vi "Camera.v3.vi"() -> ()   [LabVIEW 2015]
uses:
  Camera Properties.ctl
  Microscope Settings.ctl
  CameraState.ctl
  ModeEnum.ctl
  Stack_State.ctl
  Stack Track.ctl
  CameraControlTypeDef.ctl
  <vilib>/DAQmx/write.llb/DAQmx Write (Analog 1D Wfm NChan NSamp).vi
  <vilib>/DAQmx/create/channels.llb/DAQmx Create Channel (AO-Voltage-Basic).vi
  <vilib>/Waveform/WDTOps.llb/WDT Number of Waveform Samples DBL.vi
  <vilib>/DAQmx/configure/timing.llb/DAQmx Timing (Sample Clock).vi
  <vilib>/DAQmx/miscellaneous.llb/DAQmx Fill In Error Info.vi
  <vilib>/vision/NI_Vision_Development_Module.lvlib
  <vilib>/DAQmx/write.llb/DAQmx Write (Digital 1D Wfm NChan NSamp).vi
panel:
  out "Relax/ms":dbl
  out "Exposure/ms":dbl
  in  "Tab Control":enum32{"Camera Settings", "Recording"}(tab)
  in  "Microscope Settings":T1={"Mode"=enum."XY", {"Scanning Mode"=12.0, "Slit Width /%"=5.0}, "Piezo Position /um"=0.0, "Exposure/ms"=40.0, "Samples per millisecond"=100.0, "Relax/ms"=10.0, "Readout Direction"=2.0, "Trigger Source"=2.0} {"Trigger Source" items=["Internal"=1.0, "External"=2.0]; "Readout Direction" items=["Forward"=1.0, "Backward"=2.0]; "?"."Scanning Mode" items=["Full Frame"=1.0, "Slit Scanning"=12.0]}
  in  "Scan":bool
  in  "Scan Continuously":bool
  out "error IO":errorcluster
  in  "V Height":dbl=2048.0 min=4.0 max=2048.0 step=4.0
  in  "V Offset":dbl min=0.0 max=0.0 step=4.0
  in  "H Offset":dbl min=0.0 max=0.0 step=4.0
  in  "H Width":dbl min=4.0 max=2048.0 step=4.0
  in  "Advanced DCAM Controls":i32(listbox) caption="Multicolumn Listbox"
  in  "Properties":T2=4211904 items=["SENSOR MODE"=4212128, "CCD MODE"=4212384, "READOUT MODE"=4211872, "ACTIVE VIEW INDEX"=4343136, "BITS PER CHANNEL"=4342976, "IMAGE PIXEL TYPE"=4343296, "BINNING"=4215968, "EXPOSURE TIME"=2049184, "CONTRAST GAIN"=3163312, "CONTRAST OFFSET"=3163328, "LIGHT MODE"=2114720, "SENSITIVITY"=2114992, "PHOTON IMAGING MODE"=2115200, "HIGH DYNAMIC RANGE MODE"=3163360, "WHITE BALANCE"=3163568, "TEMPERATURE"=2115232, "TEMPERATURE TARGET"=2115264, "SENSOR COOLER FAN"=2115296, "LINEBUNDLE HEIGHT"=4212192, "MECHANICAL SHUTTER"=2115488, "BACK FOCUS POSITION"=8422304, "TRIGGER CONNECTOR"=1066432, "TRIGGER SOURCE"=1066144, "OUTPUT TRIGGER SOURCE"=1852576, "TRIGGER GLOBAL EXPOSURE"=2049680, "FIRST TRIGGER BEHAVIOR"=2049696, "CHANNEL SYNC"=1852352, "READOUT DIRECTION"=4211904, "PRE HSYNC COUNT"=1852704, "INTERNAL LINE SPEED"=4191408, "INTERNAL LINE INVERVAL"=4191424]
  out "Waves":waveform(dbl)[](graph)
  out "Image":T3(plugin-control)
  out "Histogram":T4(graph)
  in  "stop":bool
  in  "Calibration":bool
  in  "MultiD Scan":bool
  in  "Stage Controller":bool
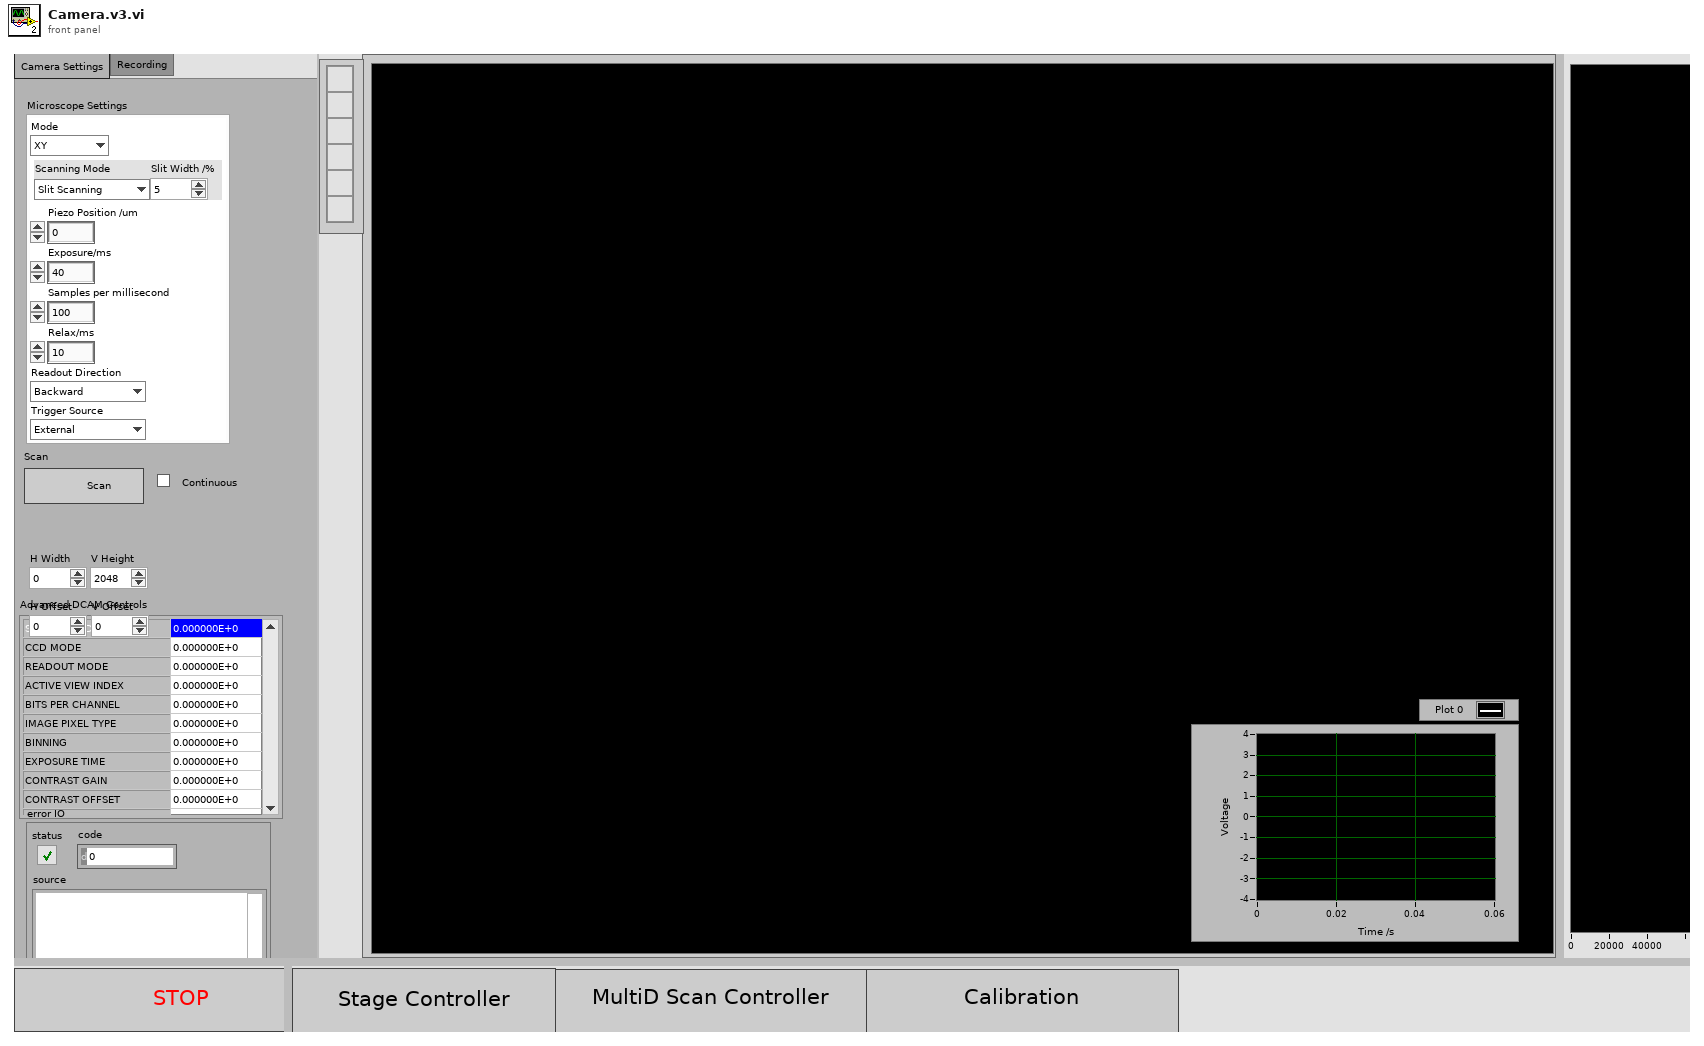
[diagram p1: front panel]
types:
  T1 = typedef "Microscope Settings.ctl" = cluster{"Mode":enum16{"X", "XY", "XYZ", "XYZT", "XYZC"}, cluster{"Scanning Mode":dbl, "Slit Width /%":dbl}, "Piezo Position /um":dbl, "Exposure/ms":dbl, "Samples per millisecond":dbl, "Relax/ms":dbl, "Readout Direction":dbl, "Trigger Source":dbl}
  T2 = typedef "Camera Properties.ctl" = u32
  T3 = typedef "IMAQ Image.ctl" = refnum<image>
  T4 = cluster{"Starting Value":sgl, "Incremental Value":sgl, "Histogram":u32[]}
  T5 = typedef "ModeEnum.ctl" = enum16{"Idle", "generateWaves", "runWaves", "stop"}
  T6 = cluster{"height":u32, "width":u32, "datatype":u32}
  T7 = typedef "CameraState.ctl" = enum16{"init", "active", "deinit"}
  T8 = typedef "CameraControlTypeDef.ctl" = enum16{"IntervalLineInt", "Ram Record", "HardDisk Record", "Disengage Update", "Update", "Idle", "ROI", "Binning", "Scan Mode", "Trigger Mode", "Readout Mode", "Readout Direction", "Preview", "ROIWindow", "Trigger Source"}
  T9 = typedef "Stack_State.ctl" = cluster{"State":T10, "Stack Number":i32, "Image":u16[][], "Stacks":i32}
  T10 = typedef "Stack Track.ctl" = enum16{"Idle", "Display", "Start Sequence", "Read Disk", "STOP", "Collecting", "End"}
  T11 = typedef "Image Type" = u32
  T12 = cluster{"Value":i32, "Minimum":i32, "Maximum":i32, "Increment":i32}
  T13 = cluster{"Minimum":i32, "Maximum":i32, "Increment":i32}
  T14 = cluster{"State":T10, "Timeout":i32, "Data 16":u16[][], "Timeout":i32}
  T15 = cluster{"Enum":T8, "Trigger Source":dbl, "timeout in ms (-1)":i32}
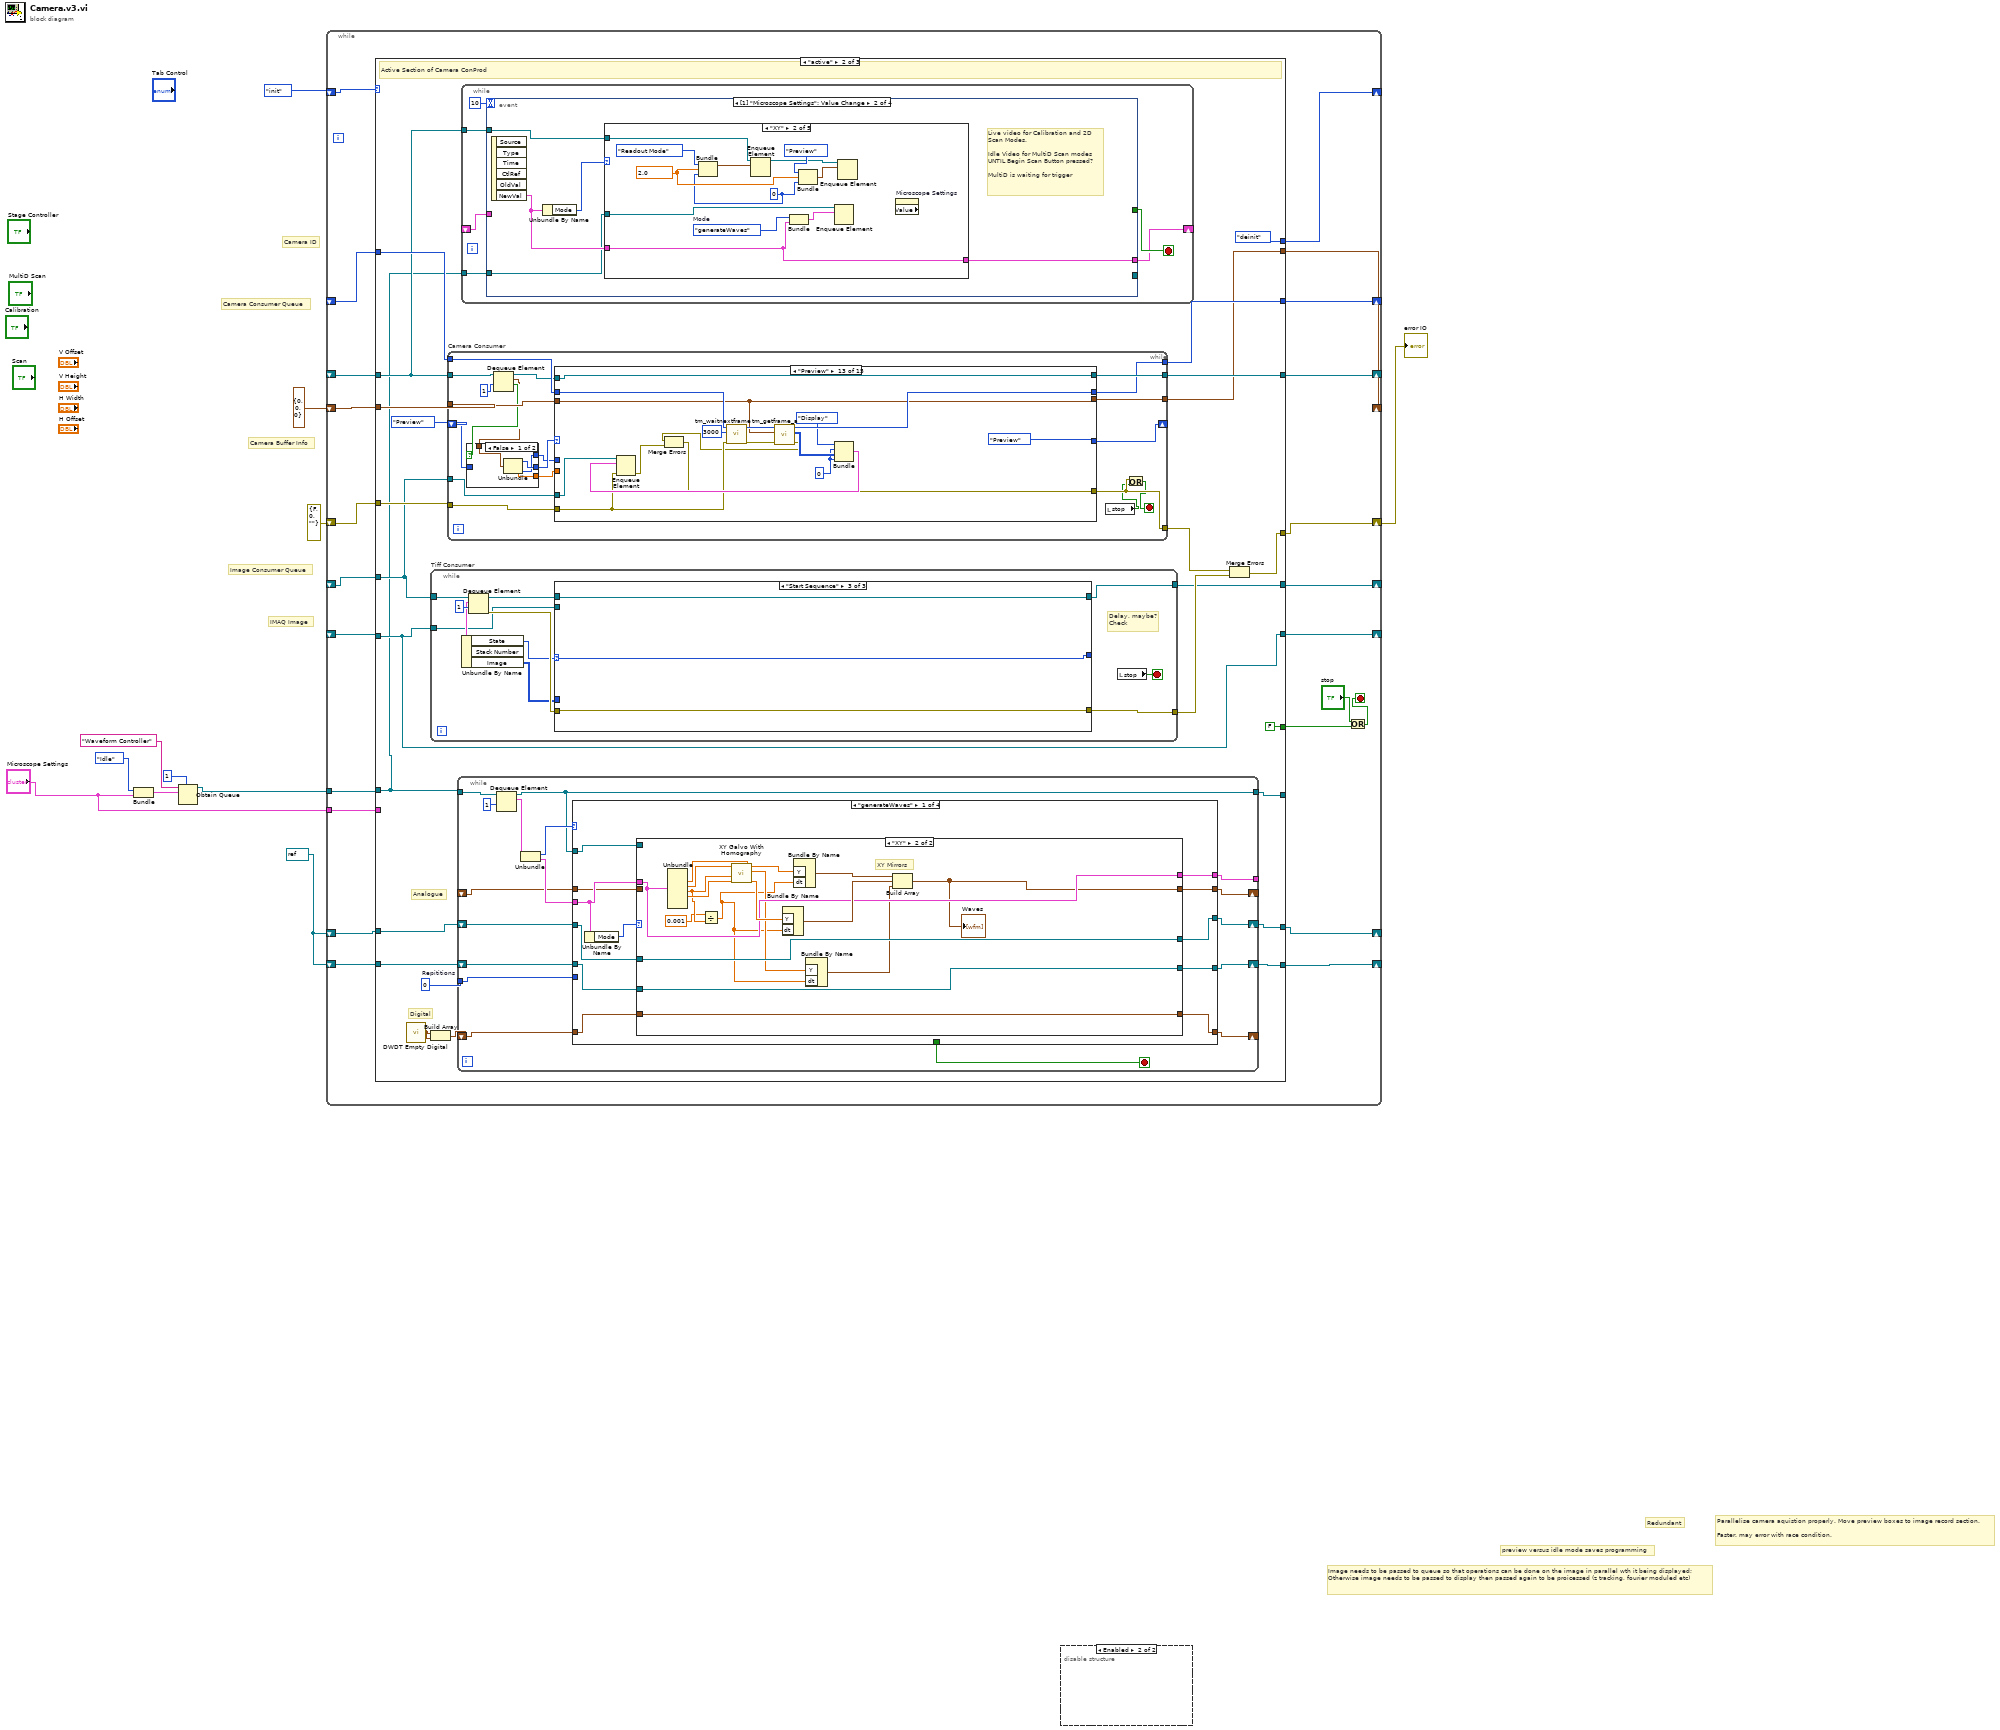
[diagram p0: block diagram]
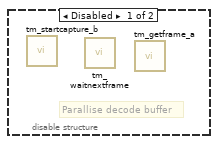
[diagram p2: hidden frame]
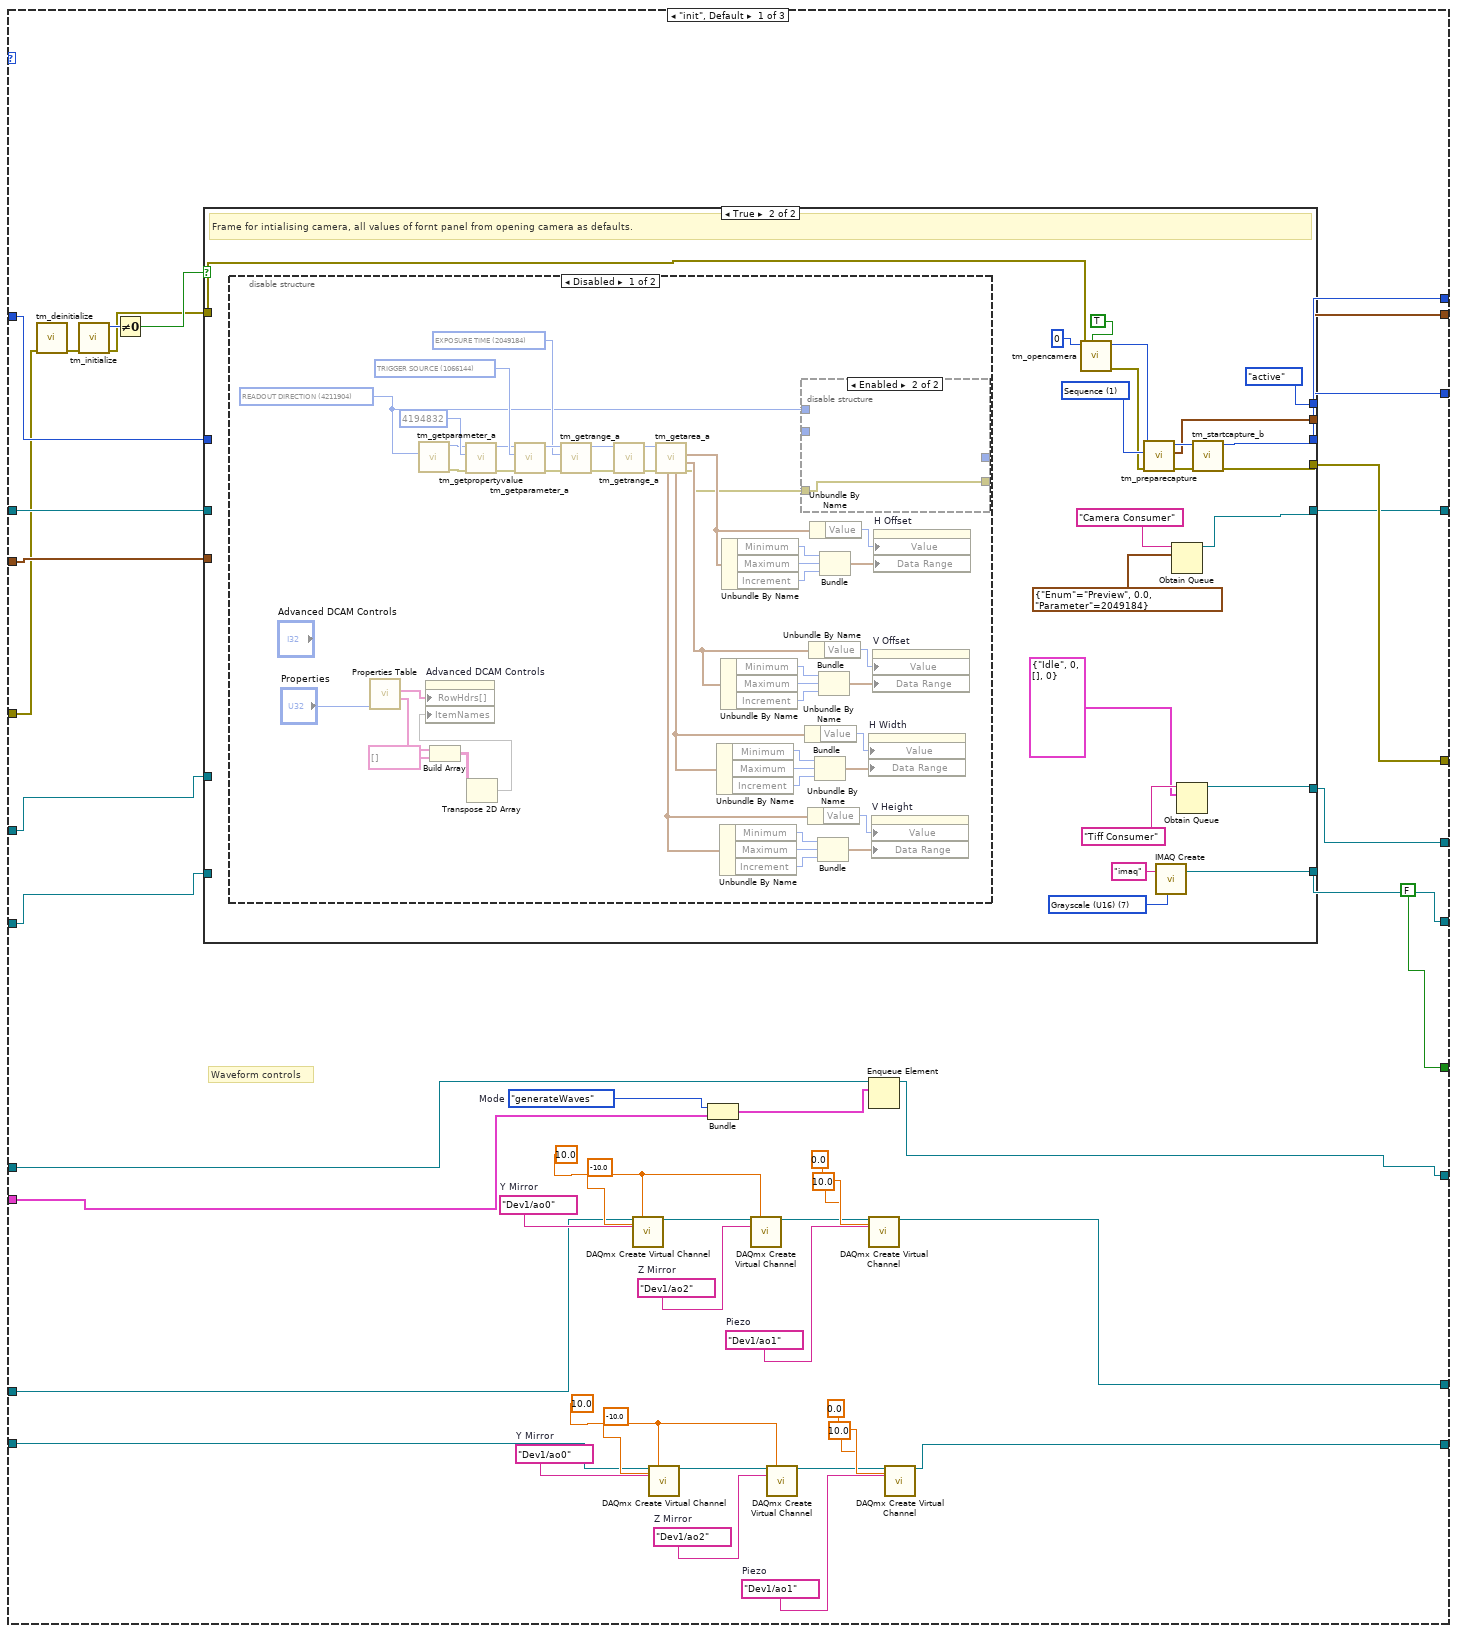
[diagram p3: hidden frame]
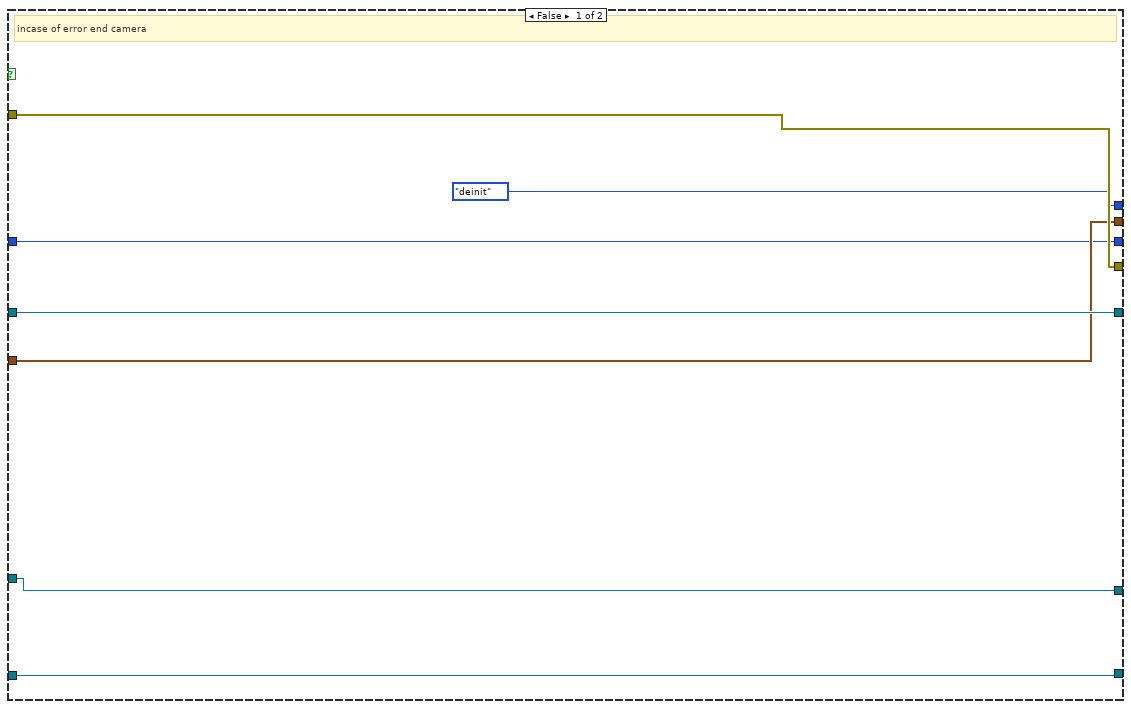
[diagram p4: hidden frame]
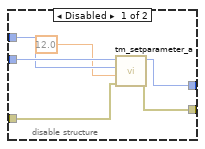
[diagram p5: hidden frame]
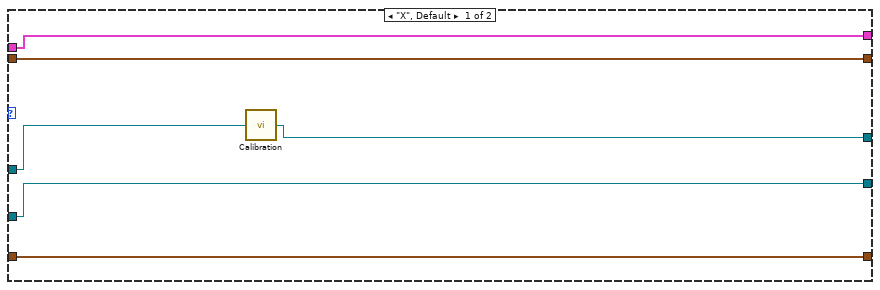
[diagram p7: hidden frame]
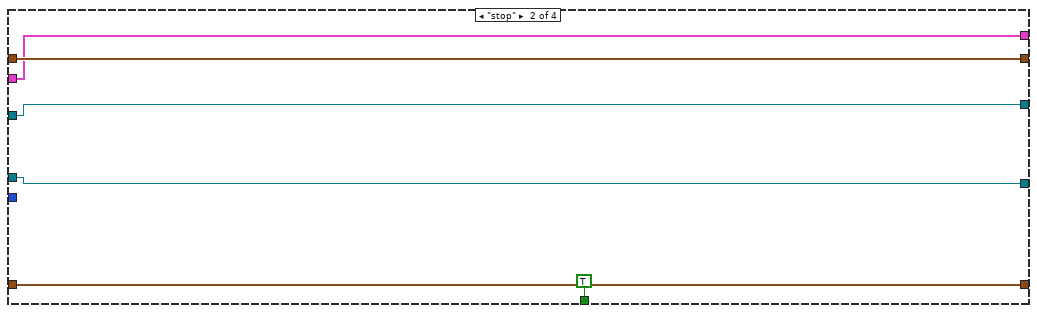
[diagram p8: hidden frame]
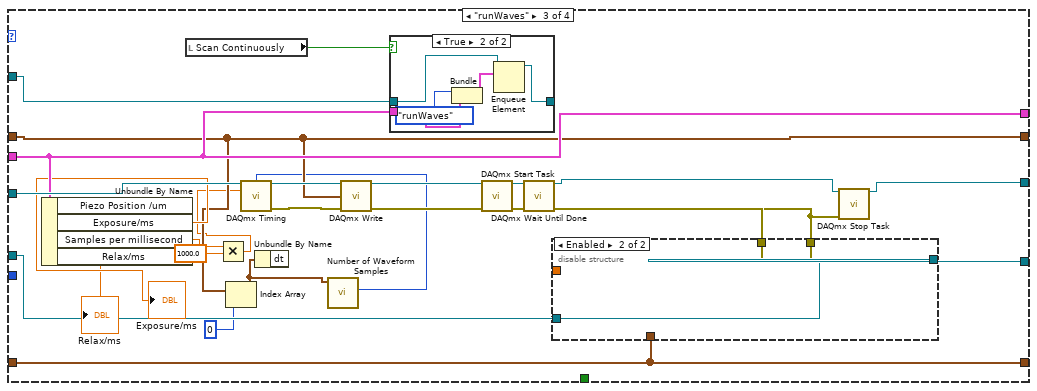
[diagram p9: hidden frame]
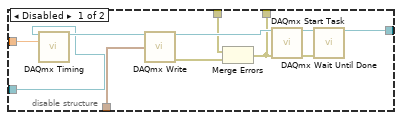
[diagram p10: hidden frame]
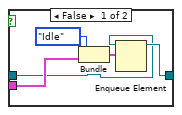
[diagram p11: hidden frame]
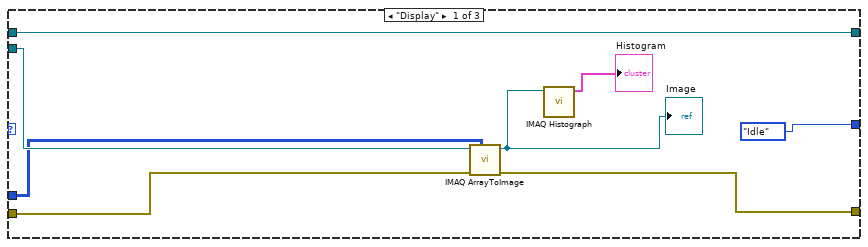
[diagram p13: hidden frame]
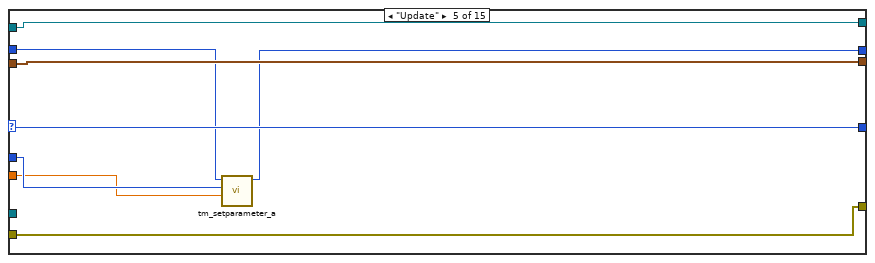
[diagram p20: hidden frame]
diagram:
  w8 = refnum<k21> refnum ("Mirror Z 2")
  # "IMAQ Image"
  # "Camera Buffer Info"
  # "Image needs to be passed to queue so that operations can be done on the image in parallel wth it being displayed;\nOtherwise image needs to be passed to display then passed again to be proicessed (z tracking, fourier moduled etc)"
  # "preview versus idle mode saves programming"
  # "Parallelise camera aquistion properly. Move preview boxes to image record section.\n\nFaster. may error with race condition."
  # "Redundant"
  # "Image Consumer Queue"
  # "Camera Consumer Queue"
  # "Camera ID"
  n1 = Bundle("Mode"=ModeEnum."Idle", "Microscope Settings"="Microscope Settings") -> (w5:cluster{"Mode":T5, "Microscope Settings":T1})  [unwired: 1 in]
  n2 = Obtain Queue(max queue size (-1, unlimited)=1, name (unnamed)="Waveform Controller", element data type=w5) -> (queue out=w1:refnum<queue>)  [unwired: 2 in, 2 out]
  n3 = while {
    shift-right: [w34] -> _
    shift-left: CameraState."init" -> [w33]
    shift-right: [w32] -> _
    shift-left: _ -> [w31]
    shift-right: [w30] -> w10
    shift-left: errorcluster {"status"=FALSE, "code"=0, "source"=""} ("error IO") -> [w29]
    shift-right: [w27] -> _
    shift-left: _ -> [w26]
    shift-right: [w28] -> _
    shift-left: _ -> [w25]
    shift-right: [w21] -> _
    shift-left: T6 {"height"=0, "width"=0, "datatype"=0} ("Buffer Info") -> [w20]
    shift-right: [w19] -> _
    shift-left: _ -> [w18]
    shift-right: [w17] -> _
    shift-left: w8 -> [w16]
    shift-right: [w14] -> _
    shift-left: w8 -> [w15]
    tunnel: "Microscope Settings" -> [w13]
    tunnel: w1 -> [w12]
    stop <- w23 stop-if-true
    n4 = case shown="\"active\"" w33 {
      tunnel: [w75 CameraState."deinit" CameraState."init"] -> w34
      tunnel: [w74 w183 w507] -> w32
      tunnel: w31 -> [w52 w184 w507]
      tunnel: [w73 w182 w510] -> w30
      tunnel: w29 -> [w51 w176 w511]
      tunnel: [w72 w179 w494] -> w28
      tunnel: [w71 w178 w490] -> w27
      tunnel: w26 -> [w69 w171 w490]
      tunnel: w25 -> [w70 w169 w494]
      tunnel: [FALSE ("stop") FALSE ("stop") TRUE ("stop")] -> w22
      tunnel: [w67 w174 w504] -> w21
      tunnel: w20 -> [w66 w173 w504]
      tunnel: w18 -> [w64 w170 w503]
      tunnel: [w65 w170 w503] -> w19
      tunnel: w12 -> [w38 w161 w489]
      tunnel: [w56 w162 w501] -> w17
      tunnel: w16 -> [w53 w165 w501]
      tunnel: w15 -> [w41 w164 w499]
      tunnel: [w40 w163 w499] -> w14
      tunnel: [w39 w160 w489] -> _
      tunnel: w13 -> [w37 _ _]
      frame "init", Default {
        w35 = ModeEnum."generateWaves"  # Mode
        w46 = tag "Dev1/ao1"  # Piezo
        w47 = tag "Dev1/ao2"  # Z Mirror
        w48 = tag "Dev1/ao0"  # Y Mirror
        w50 = 10.0 ("maximum value")
        w59 = tag "Dev1/ao1"  # Piezo
        w60 = tag "Dev1/ao2"  # Z Mirror
        w61 = tag "Dev1/ao0"  # Y Mirror
        w63 = 10.0 ("maximum value")
        # "Waveform controls"
        n5 = call "tm_deinitialize.vi"("error in (no error)"=w51) -> ("error out"=w79:errorcluster)  [unwired: 10 in]
        n6 = call "tm_initialize.vi"("error in (no error)"=w79) -> ("error out"=w76:errorcluster, "Number Of Cameras"=w78:u32)  [unwired: 7 in, 2 out]
        n7 = Not Equal To 0?(x=w78) -> (x != 0?=w77:bool)
        n8 = case shown="True" w77 {
          tunnel: w76 -> [w86 w105]
          tunnel: [CameraState."deinit" CameraState."active"] -> w75
          tunnel: [w86 w102] -> w73
          tunnel: [w81 w100] -> w74
          tunnel: [w84 w87] -> w72
          tunnel: [w83 w97] -> w71
          tunnel: w70 -> [w84 _]
          tunnel: w69 -> [w83 _]
          tunnel: [w82 w95] -> w67
          tunnel: w66 -> [w82 _]
          tunnel: w52 -> [w81 _]
          tunnel: [w80 w92] -> w65
          tunnel: w64 -> [w80 _]
          frame False {
            # "incase of error end camera"
          }
          frame True {
            w94 = T11 7 items=["Grayscale (U8)", "Grayscale (I16)", "Grayscale (SGL)", "Complex (CSG)", "RGB (U32)", "HSL (U32)", "RGB (U64)", "Grayscale (U16)"] ("Image Type")
            w104 = 1 items=["Snap", "Sequence"] ("Capture mode")
            # "Frame for intialising camera, all values of fornt panel from opening camera as defaults."
            n9 = disable-structure shown="Disabled" {
              frame Disabled {
                w149 = u32 2049184 items=["SENSOR MODE"=4212128, "CCD MODE"=4212384, "READOUT MODE"=4211872, "ACTIVE VIEW INDEX"=4343136, "BITS PER CHANNEL"=4342976, "IMAGE PIXEL TYPE"=4343296, "BINNING"=4215968, "EXPOSURE TIME"=2049184, "CONTRAST GAIN"=3163312, "CONTRAST OFFSET"=3163328, "LIGHT MODE"=2114720, "SENSITIVITY"=2114992, "PHOTON IMAGING MODE"=2115200, "HIGH DYNAMIC RANGE MODE"=3163360, "WHITE BALANCE"=3163568, "TEMPERATURE"=2115232, "TEMPERATURE TARGET"=2115264, "SENSOR COOLER FAN"=2115296, "LINEBUNDLE HEIGHT"=4212192, "MECHANICAL SHUTTER"=2115488, "BACK FOCUS POSITION"=8422304, "TRIGGER CONNECTOR"=1066432, "TRIGGER SOURCE"=1066144, "OUTPUT TRIGGER SOURCE"=1852576, "TRIGGER GLOBAL EXPOSURE"=2049680, "FIRST TRIGGER BEHAVIOR"=2049696, "CHANNEL SYNC"=1852352, "READOUT DIRECTION"=4211904, "PRE HSYNC COUNT"=1852704, "INTERNAL LINE SPEED"=4191408, "INTERNAL LINE INVERVAL"=4191424] ("Parameter")
                w109 = T2 4211904 items=["SENSOR MODE"=4212128, "CCD MODE"=4212384, "READOUT MODE"=4211872, "ACTIVE VIEW INDEX"=4343136, "BITS PER CHANNEL"=4342976, "IMAGE PIXEL TYPE"=4343296, "BINNING"=4215968, "EXPOSURE TIME"=2049184, "CONTRAST GAIN"=3163312, "CONTRAST OFFSET"=3163328, "LIGHT MODE"=2114720, "SENSITIVITY"=2114992, "PHOTON IMAGING MODE"=2115200, "HIGH DYNAMIC RANGE MODE"=3163360, "WHITE BALANCE"=3163568, "TEMPERATURE"=2115232, "TEMPERATURE TARGET"=2115264, "SENSOR COOLER FAN"=2115296, "LINEBUNDLE HEIGHT"=4212192, "MECHANICAL SHUTTER"=2115488, "BACK FOCUS POSITION"=8422304, "TRIGGER CONNECTOR"=1066432, "TRIGGER SOURCE"=1066144, "OUTPUT TRIGGER SOURCE"=1852576, "TRIGGER GLOBAL EXPOSURE"=2049680, "FIRST TRIGGER BEHAVIOR"=2049696, "CHANNEL SYNC"=1852352, "READOUT DIRECTION"=4211904, "PRE HSYNC COUNT"=1852704, "INTERNAL LINE SPEED"=4191408, "INTERNAL LINE INVERVAL"=4191424] ("Parameter")
                w152 = u32 1066144 items=["SENSOR MODE"=4212128, "CCD MODE"=4212384, "READOUT MODE"=4211872, "ACTIVE VIEW INDEX"=4343136, "BITS PER CHANNEL"=4342976, "IMAGE PIXEL TYPE"=4343296, "BINNING"=4215968, "EXPOSURE TIME"=2049184, "CONTRAST GAIN"=3163312, "CONTRAST OFFSET"=3163328, "LIGHT MODE"=2114720, "SENSITIVITY"=2114992, "PHOTON IMAGING MODE"=2115200, "HIGH DYNAMIC RANGE MODE"=3163360, "WHITE BALANCE"=3163568, "TEMPERATURE"=2115232, "TEMPERATURE TARGET"=2115264, "SENSOR COOLER FAN"=2115296, "LINEBUNDLE HEIGHT"=4212192, "MECHANICAL SHUTTER"=2115488, "BACK FOCUS POSITION"=8422304, "TRIGGER CONNECTOR"=1066432, "TRIGGER SOURCE"=1066144, "OUTPUT TRIGGER SOURCE"=1852576, "TRIGGER GLOBAL EXPOSURE"=2049680, "FIRST TRIGGER BEHAVIOR"=2049696, "CHANNEL SYNC"=1852352, "READOUT DIRECTION"=4211904, "PRE HSYNC COUNT"=1852704, "INTERNAL LINE SPEED"=4191408, "INTERNAL LINE INVERVAL"=4191424] ("Parameter")
                n10 = call "Properties Table.vi"("Properties"="Properties") -> ("Value Stirngs Out"=w114:string[], "Row Headers"=w115:string[])  [unwired: 4 in, 2 out]
                n11 = call "tm_getparameter_a.vi"("Parameter"=w109) -> ("error out"=w141:errorcluster, "Handle out"=w143:u32)  [unwired: 8 in, 1 out]
                n12 = Build Array(w114, string[] [] ("element")) -> (w112:string[][])
                n13 = call "tm_getpropertyvalue.vi"("error in (no error)"=w141, "Property ID"=u32 4194832, "Handle in"=w143) -> ("error out"=w142:errorcluster, "Handle out"=w108:u32)  [unwired: 6 in, 1 out]
                n14 = Transpose 2D Array(2D array=w112) -> (transposed array=w111:string[][])
                n15 = property on="Advanced DCAM Controls" class="MCListbox (strict)"("RowHdrs[]"=w115, "ItemNames"=w111) -> ()  [unwired: 2 in, 2 out]
                n16 = call "tm_getparameter_a.vi"("error in (no error)"=w142, "Parameter"=w152, "Handle in"=w108) -> ("error out"=w150:errorcluster, "Handle out"=w151:u32)  [unwired: 6 in, 1 out]
                n17 = call "tm_getrange_a.vi"("error in (no error)"=w150, "Parameter"=w149, "Handle in"=w151) -> ("error out"=w147:errorcluster, "Handle out"=w148:u32)  [unwired: 2 in, 5 out]
                n18 = call "tm_getrange_a.vi"("error in (no error)"=w147, "Handle in"=w148) -> ("error out"=w146:errorcluster, "Handle out"=w145:u32)  [unwired: 3 in, 5 out]
                n19 = call "tm_getarea_a.vi"("error in (no error)"=w146, "Handle in"=w145) -> ("error out"=w110:errorcluster, "V Offset"=w117:T12, "H Offset"=w140:T12, "H Width"=w118:T12, "V Width"=w119:T12)  [unwired: 4 in, 1 out]
                n20 = Unbundle By Name(w118) -> ("Minimum"=w129:i32, "Maximum"=w128:i32, "Increment"=w127:i32)
                n21 = Unbundle By Name(w119) -> ("Minimum"=w120:i32, "Maximum"=w121:i32, "Increment"=w122:i32)
                n22 = Unbundle By Name(w117) -> ("Minimum"=w130:i32, "Maximum"=w131:i32, "Increment"=w132:i32)
                n23 = Unbundle By Name(w140) -> ("Minimum"=w139:i32, "Maximum"=w138:i32, "Increment"=w137:i32)
                n24 = disable-structure shown="Enabled" {
                  disable-tunnel: _ -> [w158 _]
                  disable-tunnel: [w157 _] -> _
                  disable-tunnel: w110 -> [w156 w159]
                  disable-tunnel: [w155 w159] -> _
                  disable-tunnel: w109 -> [w154 _]
                  frame Disabled {
                    n25 = call "tm_setparameter_a.vi"("error in (no error)"=w156, "Value in"=12.0, "Parameter"=w154, "Handle in"=w158) -> ("error out"=w155:errorcluster, "Handle out"=w157:u32)  [unwired: 6 in]
                  }
                  frame Enabled {
                  }
                }
                n26 = Unbundle By Name(w118) -> ("Value"=w125:i32)
                n27 = Unbundle By Name(w119) -> ("Value"=w124:i32)
                n28 = Unbundle By Name(w117) -> ("Value"=w134:i32)
                n29 = Unbundle By Name(w140) -> ("Value"=w135:i32)
                n30 = Bundle("Minimum"=w129, "Maximum"=w128, "Increment"=w127) -> (w126:T13)  [unwired: 1 in]
                n31 = Bundle("Minimum"=w120, "Maximum"=w121, "Increment"=w122) -> (w123:T13)  [unwired: 1 in]
                n32 = Bundle("Minimum"=w130, "Maximum"=w131, "Increment"=w132) -> (w133:T13)  [unwired: 1 in]
                n33 = Bundle("Minimum"=w139, "Maximum"=w138, "Increment"=w137) -> (w136:T13)  [unwired: 1 in]
                n34 = property on="H Width" class="DigNum (strict)"("Value"=w125, "Data Range"=w126) -> ()  [unwired: 2 in, 2 out]
                n35 = property on="V Height" class="DigNum (strict)"("Value"=w124, "Data Range"=w123) -> ()  [unwired: 2 in, 2 out]
                n36 = property on="V Offset" class="DigNum (strict)"("Value"=w134, "Data Range"=w133) -> ()  [unwired: 2 in, 2 out]
                n37 = property on="H Offset" class="DigNum (strict)"("Value"=w135, "Data Range"=w136) -> ()  [unwired: 2 in, 2 out]
              }
              frame Enabled {
              }
            }
            n38 = call "tm_opencamera.vi"("Force Open"=TRUE, "error in (no error)"=w105, "Camera Index"=u32 0) -> ("error out"=w89:errorcluster, "Handle out"=w88:u32)  [unwired: 6 in, 1 out]
            n39 = call "tm_preparecapture.vi"("error in (no error)"=w89, "Capture mode"=w104, "Handle in"=w88) -> ("error out"=w103:errorcluster, "Buffer Info"=w95:T6, "Handle out"=w101:u32)  [unwired: 5 in, 1 out]
            n40 = call "IMAQ Create"("Image Name"="imaq", "Image Type"=w94) -> ("New Image"=w92:T3)  [unwired: 3 in, 1 out]
            n41 = Obtain Queue(name (unnamed)="Camera Consumer", element data type=cluster{"Enum":T8, dbl, "Parameter":u32} {"Enum"=enum."Preview", 0.0, "Parameter"=2049184}) -> (queue out=w87:refnum<queue>)  [unwired: 3 in, 2 out]
            n42 = Obtain Queue(name (unnamed)="Tiff Consumer", element data type=T9 {"State"=enum."Idle", "Stack Number"=0, "Image"=[], "Stacks"=0} ("input cluster")) -> (queue out=w97:refnum<queue>)  [unwired: 3 in, 2 out]
            n43 = call "tm_startcapture_b.vi"("error in (no error)"=w103, "Handle in"=w101) -> ("error out"=w102:errorcluster, "Handle out"=w100:u32)  [unwired: 8 in]
          }
        }
        n44 = call-poly <vilib>:"DAQmx Create Virtual Channel.vi"("task in"=w53, "maximum value"=w63, "minimum value"=-10.0, "physical channels"=w61) -> ("task out"=w55:refnum<k21>)  [unwired: 10 in, 1 out]
        n45 = call-poly <vilib>:"DAQmx Create Virtual Channel.vi"("task in"=w41, "maximum value"=w50, "minimum value"=-10.0, "physical channels"=w48) -> ("task out"=w43:refnum<k21>)  [unwired: 10 in, 1 out]
        n46 = Bundle("Mode"=w35, "Microscope Settings"=w37) -> (w36:cluster{"Mode":T5, "Microscope Settings":T1})  [unwired: 1 in]
        n47 = call-poly <vilib>:"DAQmx Create Virtual Channel.vi"("task in"=w55, "maximum value"=w63, "physical channels"=w60) -> ("task out"=w54:refnum<k21>)  [unwired: 11 in, 1 out]
        n48 = call-poly <vilib>:"DAQmx Create Virtual Channel.vi"("task in"=w43, "maximum value"=w50, "physical channels"=w47) -> ("task out"=w42:refnum<k21>)  [unwired: 11 in, 1 out]
        n49 = Enqueue Element(queue=w38, element=w36) -> (queue out=w39:refnum<queue>)  [unwired: 2 in, 2 out]
        n50 = call-poly <vilib>:"DAQmx Create Virtual Channel.vi"("task in"=w54, "maximum value"=10.0 ("minimum value"), "minimum value"=0.0 ("maximum value"), "physical channels"=w59) -> ("task out"=w56:refnum<k21>)  [unwired: 10 in, 1 out]
        n51 = call-poly <vilib>:"DAQmx Create Virtual Channel.vi"("task in"=w42, "maximum value"=10.0 ("minimum value"), "minimum value"=0.0 ("maximum value"), "physical channels"=w46) -> ("task out"=w40:refnum<k21>)  [unwired: 10 in, 1 out]
      }
      frame "active" {
        w168 = 0  # Repititions
        # "Digital"
        # "Analogue"
        # "Active Section of Camera ConProd"
        n52 = call <vilib>:"DWDT Empty Digital.vi"() -> ("digital waveform out"=w166:digitalwaveform)  [unwired: 5 in]
        n53 = while "Tiff Consumer" {
          tunnel: [w299] -> w181
          tunnel: [w302] -> w178
          tunnel: w171 -> [w304]
          tunnel: w170 -> [w296]
          stop <- w306 stop-if-true
          # "Delay, maybe?\nCheck"
          n54 = Dequeue Element(queue=w304, timeout in ms (-1)=1) -> (queue out=w301:refnum<queue>, element=w303:T9, error out=w300:errorcluster)  [unwired: 1 in, 1 out]
          n55 = Unbundle By Name(w303) -> ("State"=w297:T10, "Image"=w298:u16[][])  [unwired: 1 out]
          n56 = case shown="\"Start Sequence\"" w297 {
            selector: w297 -> [_ w317 w318]
            tunnel: [w314 w316 w319] -> w302
            tunnel: w301 -> [w314 w316 w319]
            tunnel: [Stack_Track."Idle" ("State") w317 w318] -> _
            tunnel: w298 -> [w309 _ _]
            tunnel: w296 -> [w313 _ _]
            tunnel: w300 -> [w312 w315 w320]
            tunnel: [w311 w315 w320] -> w299
            frame "Display" {
              n57 = call "IMAQ ArrayToImage"("Image Pixels (U16)"=w309, "error in (no error)"=w312, "Image"=w313) -> ("error out"=w311:errorcluster, "Image Out"=w308:T3)  [unwired: 7 in]
              "Image" <- w308
              n58 = call "IMAQ Histograph"("Image"=w308) -> ("Histogram Graph"=→"Histogram":T4)  [unwired: 7 in, 3 out]
            }
            frame "Idle", Default {
            }
            frame "Start Sequence" {
            }
          }
          n59 = local read "stop"() -> (w306:bool)
        }
        n60 = Build Array(w166, w166) -> (w167:digitalwaveform[])
        n61 = while "Camera Consumer" {
          tunnel: w176 -> [w339]
          tunnel: w184 -> [w337]
          tunnel: [w336] -> w183
          tunnel: [w323] -> w180
          tunnel: w169 -> [w332]
          tunnel: [w340] -> w179
          shift-right: [w338] -> _
          shift-left: CameraControlTypeDef."Preview" ("Enum") -> [w328]
          tunnel: [w335] -> w174
          tunnel: w173 -> [w334]
          tunnel: w171 -> [w327]
          stop <- w321 stop-if-true
          n62 = Dequeue Element(queue=w332, timeout in ms (-1)=1) -> (queue out=w331:refnum<queue>, element=w326:cluster{"Enum":T8, dbl, "Parameter":u32}, timed out?=w330:bool)  [unwired: 1 in, 1 out]
          n63 = case shown="False" w330 {
            tunnel: [w343 w345] -> w329
            tunnel: w328 -> [_ w345]
            tunnel: w326 -> [w344 _]
            tunnel: [w342 _] -> w325
            tunnel: [w341 w345] -> w324
            frame False {
              n64 = Unbundle(w344) -> ("Enum"=w343:T8, w342:dbl, "Parameter"=w341:u32)
            }
            frame True {
            }
          }
          n65 = case shown="\"Preview\"" w329 {
            selector: w329 -> [w349 w354 w359 w364 w372 w377 w382 w387 w392 w397 w402 w407 _ w428 _]
            tunnel: w331 -> [w348 w355 w360 w365 w373 w378 w383 w388 w393 w398 w403 w408 w425 w430 w435]
            tunnel: [w348 w355 w360 w365 w373 w378 w383 w388 w393 w398 w403 w408 w425 w430 w435] -> w340
            tunnel: w339 -> [w350 w353 w358 w363 w371 w376 w381 w386 w391 w396 w401 w406 w412 w427 w433]
            tunnel: [w350 w353 w358 w363 w371 w376 w381 w386 w391 w396 w401 w406 w409 w427 w433] -> w323
            tunnel: [w349 w354 w359 w364 w372 w377 w382 w387 w392 w397 w402 w407 CameraControlTypeDef."Preview" ("Enum") w428 CameraControlTypeDef."Preview" ("Enum")] -> w338
            tunnel: w337 -> [w347 w352 w357 w362 w369 w375 w380 w385 w390 w395 w400 w405 w423 w429 w434]
            tunnel: [w347 w352 w357 w362 w368 w375 w380 w385 w390 w395 w400 w405 w421 w429 w434] -> w336
            tunnel: [w346 w351 w356 w361 w370 w374 w379 w384 w389 w394 w399 w404 w418 w426 w432] -> w335
            tunnel: w334 -> [w346 w351 w356 w361 w370 w374 w379 w384 w389 w394 w399 w404 w418 w426 w432]
            tunnel: w327 -> [_ _ _ _ _ _ _ _ _ _ _ _ w417 _ _]
            tunnel: w325 -> [_ _ _ _ w366 _ _ _ _ _ _ _ _ _ _]
            tunnel: w324 -> [_ _ _ _ w367 _ _ _ _ _ _ _ _ _ _]
            frame "IntervalLineInt" {
            }
            frame "Ram Record" {
            }
            frame "HardDisk Record" {
            }
            frame "Disengage Update" {
            }
            frame "Update" {
              n66 = call "tm_setparameter_a.vi"("Value in"=w366, "Parameter"=w367, "Handle in"=w369) -> ("Handle out"=w368:u32)  [unwired: 7 in, 1 out]
            }
            frame "Idle", Default {
            }
            frame "ROI" {
            }
            frame "Binning" {
            }
            frame "Scan Mode" {
            }
            frame "Trigger Mode" {
            }
            frame "Readout Mode" {
            }
            frame "Readout Direction" {
            }
            frame "Preview" {
              w414 = 0 ("Timeout")
              n67 = call "tm_waitnextframe.vi"("error in (no error)"=w412, "Timeout"=3000, "Handle in"=w423) -> ("error out"=w420:errorcluster, "Handle out"=w422:u32)  [unwired: 5 in, 2 out]
              n68 = call "tm_getframe_a.vi"("error in (no error)"=w420, "Buffer Info"=w418, "Handle in"=w422) -> ("error out"=w410:errorcluster, "Data 16"=w415:u16[][], "Handle out"=w421:u32)  [unwired: 4 in, 2 out]
              n69 = Bundle("State"=Stack_Track."Display", "Timeout"=w414, "Data 16"=w415, "Timeout"=w414) -> (w413:T14)  [unwired: 1 in]
              n70 = Enqueue Element(queue=w417, element=w413, error in (no error)=w412) -> (error out=w411:errorcluster)  [unwired: 1 in, 2 out]
              n71 = Merge Errors(w410, w411) -> (w409:errorcluster)
            }
            frame "ROIWindow" {
            }
            frame "Trigger Source" {
              n72 = call "tm_unpreparecapture.vi"() -> ()  [unwired: 10 in, 2 out]
              n73 = call "tm_setparameter_a.vi"() -> ()  [unwired: 10 in, 2 out]
              n74 = call "tm_preparecapture.vi"() -> ()  [unwired: 8 in, 4 out]
            }
          }
          n75 = local read "stop"() -> (w322:bool)
          n76 = Or(x=w323, y=w322) -> (x .or. y?=w321:bool)
        }
        n77 = while {
          tunnel: w161 -> [w201]
          shift-right: [w196] -> _
          shift-left: _ -> [w195]
          tunnel: w168 -> [w194]
          tunnel: [w193] -> _
          shift-right: [w189] -> w162
          shift-left: w165 -> [w188]
          shift-right: [w192] -> _
          shift-left: w167 -> [w191]
          shift-right: [w187] -> w163
          shift-left: w164 -> [w186]
          tunnel: [w185] -> w160
          stop <- w200 stop-if-true
          n78 = Dequeue Element(queue=w201, timeout in ms (-1)=1) -> (queue out=w185:refnum<queue>, element=w199:cluster{"Mode":T5, "Microscope Settings":T1})  [unwired: 1 in, 2 out]
          n79 = Unbundle(w199) -> ("Mode"=w198:T5, "Microscope Settings"=w197:T1)
          n80 = case shown="\"generateWaves\"" w198 {
            tunnel: [_ TRUE _ _] -> w200
            tunnel: w197 -> [w212 w237 w257 w291]
            tunnel: [w213 w242 w254 w295] -> w196
            tunnel: w195 -> [w204 w242 w254 w295]
            tunnel: w194 -> [_ _ _ _]
            tunnel: w185 -> [w203 _ w258 _]
            tunnel: [w202 w237 w257 w291] -> w193
            tunnel: [w208 w241 w262 w292] -> w187
            tunnel: [w206 w240 w248 w293] -> w189
            tunnel: w188 -> [w205 w240 w259 w293]
            tunnel: [w211 w239 w266 w294] -> w192
            tunnel: w191 -> [w210 w239 w266 w294]
            tunnel: w186 -> [w209 w241 w260 w292]
            frame "generateWaves" {
              n81 = Unbundle By Name(w212) -> ("Mode"=w207:enum16{"X", "XY", "XYZ", "XYZT", "XYZC"})
              n82 = case shown="\"XY\"" w207 {
                tunnel: [w219 w223] -> w213
                tunnel: w212 -> [w218 w226]
                tunnel: [w216 w229] -> w211
                tunnel: w210 -> [w216 w229]
                tunnel: w209 -> [w217 w228]
                tunnel: [w217 w228] -> w208
                tunnel: [w214 w227] -> w206
                tunnel: w205 -> [w215 w227]
                tunnel: w204 -> [w219 _]
                tunnel: w203 -> [_ _]
                tunnel: [w218 w226] -> w202
                frame "X", Default {
                  n83 = call "Calibration.vi"("Analogue In"=w215) -> ("Analogue In Out"=w214:refnum<k21>)
                }
                frame "XY" {
                  # "XY Mirrors"
                  n84 = Unbundle(w226) -> ("Piezo Position /um"=w232:dbl, "Exposure/ms"=w230:dbl, "Samples per millisecond"=w221:dbl, "Relax/ms"=w231:dbl)  [unwired: 4 out]
                  n85 = Divide(x=0.001 ("y"), y=w221) -> (x/y=w222:dbl)
                  n86 = call "XY Galvo With Homography.vi"("Piezo Position (um)"=w232, "Relax (ms)"=w231, "Samples /Millisecond"=w221, "Exposure (ms)"=w230) -> ("Z Mirror Signal"=w235:dbl[], "Piezo Signal"=w225:dbl[], "Scan Mirror Signal"=w236:dbl[])  [unwired: 2 in]
                  n87 = Bundle By Name("Y"=w235, "dt"=w222) -> (w234:waveform(dbl))  [unwired: 1 in]
                  n88 = Bundle By Name("Y"=w236, "dt"=w222) -> (w233:waveform(dbl))  [unwired: 1 in]
                  n89 = Bundle By Name("Y"=w225, "dt"=w222) -> (w224:waveform(dbl))  [unwired: 1 in]
                  n90 = Build Array(w233, w234, w224) -> (w223:waveform(dbl)[])
                  "Waves" <- w223
                }
              }
            }
            frame "stop" {
            }
            frame "runWaves" {
              n91 = Unbundle By Name(w257) -> ("Exposure/ms"=→"Exposure/ms":dbl, "Samples per millisecond"=w246:dbl, "Relax/ms"=→"Relax/ms":dbl)  [unwired: 1 out]
              n92 = local read "Scan Continuously"() -> (w243:bool)
              n93 = Multiply(x=w246, y=1000.0) -> (x*y=w244:dbl)
              n94 = Index Array(array=w254, index=0) -> (element=w252:waveform(dbl))
              n95 = Unbundle By Name(w252) -> ()  [unwired: 1 out]
              n96 = call-poly <vilib>:"Number of Waveform Samples.vi"("waveform in"=w252) -> ("number of samples"=w251:i32)  [unwired: 8 in, 2 out]
              n97 = call-poly <vilib>:"DAQmx Timing.vi"("task/channels in"=w259, "samples per channel"=w251, "rate"=w244) -> ("task out"=w267:refnum<k21>, "error out"=w250:errorcluster)  [unwired: 11 in]
              n98 = call-poly <vilib>:"DAQmx Write.vi"("task/channels in"=w267, "data"=w254, "error in"=w250) -> ("task out"=w265:refnum<k21>, "error out"=w264:errorcluster)  [unwired: 10 in, 1 out]
              n99 = case shown="True" w243 {
                tunnel: w258 -> [w282 w290]
                tunnel: [w283 w289] -> _
                tunnel: w257 -> [w284 w288]
                frame False {
                  n100 = Bundle("Mode"=ModeEnum."Idle", "Microscope Settings"=w284) -> (w285:cluster{"Mode":T5, "Microscope Settings":T1})  [unwired: 1 in]
                  n101 = Enqueue Element(queue=w282, element=w285) -> (queue out=w283:refnum<queue>)  [unwired: 2 in, 2 out]
                }
                frame True {
                  n102 = Bundle("Mode"=ModeEnum."runWaves", "Microscope Settings"=w288) -> (w287:cluster{"Mode":T5, "Microscope Settings":T1})  [unwired: 1 in]
                  n103 = Enqueue Element(queue=w290, element=w287) -> (queue out=w289:refnum<queue>)  [unwired: 2 in, 2 out]
                }
              }
              n104 = disable-structure shown="Enabled" {
                disable-tunnel: _ -> [w278 _]
                disable-tunnel: w266 -> [w276 _]
                disable-tunnel: w264 -> [w273 w279]
                disable-tunnel: [w272 w279] -> w247
                disable-tunnel: [w270 w280] -> w262
                disable-tunnel: w260 -> [w268 w280]
                frame Disabled {
                  n105 = call-poly <vilib>:"DAQmx Timing.vi"("task/channels in"=w268, "rate"=w278) -> ("task out"=w277:refnum<k21>)  [unwired: 12 in, 1 out]
                  n106 = call-poly <vilib>:"DAQmx Write.vi"("task/channels in"=w277, "data"=w276) -> ("task out"=w275:refnum<k21>, "error out"=w274:errorcluster)  [unwired: 11 in, 1 out]
                  n107 = Merge Errors(w273, w274) -> (w272:errorcluster)
                  n108 = call <vilib>:"DAQmx Start Task.vi"("task/channels in"=w275, "error in"=w272) -> ("task out"=w271:refnum<k21>, "error out"=w269:errorcluster)  [unwired: 12 in]
                  n109 = call <vilib>:"DAQmx Wait Until Done.vi"("task/channels in"=w271, "error in"=w269) -> ("task out"=w270:refnum<k21>)  [unwired: 12 in, 1 out]
                }
                frame Enabled {
                }
              }
              n110 = call <vilib>:"DAQmx Start Task.vi"("task/channels in"=w265, "error in"=w247) -> ("task out"=w263:refnum<k21>, "error out"=w261:errorcluster)  [unwired: 12 in]
              n111 = call <vilib>:"DAQmx Wait Until Done.vi"("task/channels in"=w263, "error in"=w261) -> ("task out"=w249:refnum<k21>)  [unwired: 12 in, 1 out]
              n112 = call <vilib>:"DAQmx Stop Task.vi"("task/channels in"=w249, "error in"=w247) -> ("task out"=w248:refnum<k21>)  [unwired: 12 in, 1 out]
            }
            frame "Idle", Default {
            }
          }
        }
        n113 = while {
          tunnel: w169 -> [w440]
          shift-right: [w439] -> _
          shift-left: _ -> [w438]
          tunnel: w161 -> [w436]
          stop <- w441 stop-if-true
          n114 = event shown="[1] \"Microscope Settings\": Value Change" {
            selector: _ -> [_ _ _ _]
            dyn-events: _ -> [_ _ _ _]
            timeout: 10 -> [_ _ _ _]
            tunnel: [w442 _ _ _] -> w441
            tunnel: w440 -> [_ w447 _ _]
            tunnel: [_ w444 _ w488] -> w439
            tunnel: w438 -> [_ _ w485 _]
            tunnel: [_ _ w484 _] -> _
            tunnel: w436 -> [_ w443 w483 _]
            event "stop": Value Change {
              n115 = event-data() -> ()  [unwired: 1 in, 6 out]
              n116 = local read "stop"() -> (w442:bool)
            }
            event Value Change {
              # "Live video for Calibration and 2D\nScan Modes.\n\nIdle Video for MultiD Scan modes\nUNTIL Begin Scan Button pressed?\n\nMultiD is waiting for trigger"
              n117 = event-data() -> ("NewVal"=w446:T1)  [unwired: 1 in, 5 out]
              n118 = Unbundle By Name(w446) -> ("Mode"=w445:enum16{"X", "XY", "XYZ", "XYZT", "XYZC"})
              n119 = case shown="\"XY\"" w445 {
                tunnel: w447 -> [w458 w470 w479 _ _]
                tunnel: w446 -> [w449 w461 w472 w481 w482]
                tunnel: [w449 w461 w472 w481 w482] -> w444
                tunnel: w443 -> [w448 w460 _ _ _]
                frame "X" {
                  w451 = ModeEnum."generateWaves"  # Mode
                  w452 = 0 ("timeout in ms (-1)")
                  w453 = 1.0 items=["Internal"=1.0, "External"=2.0] ("Trigger Source")
                  n120 = Bundle("Enum"=CameraControlTypeDef."Readout Mode", "Trigger Source"=w453, "timeout in ms (-1)"=w452) -> (w457:T15)  [unwired: 1 in]
                  n121 = Enqueue Element(queue=w458, element=w457) -> (queue out=w455:refnum<queue>)  [unwired: 2 in, 2 out]
                  n122 = Bundle("Enum"=CameraControlTypeDef."Preview", "Trigger Source"=w453, "timeout in ms (-1)"=w452) -> (w456:T15)  [unwired: 1 in]
                  n123 = Bundle("Mode"=w451, "NewVal"=w449) -> (w450:cluster{"Mode":T5, "NewVal":T1})  [unwired: 1 in]
                  n124 = Enqueue Element(queue=w455, element=w456) -> ()  [unwired: 2 in, 3 out]
                  n125 = Enqueue Element(queue=w448, element=w450) -> ()  [unwired: 2 in, 3 out]
                }
                frame "XY" {
                  w463 = ModeEnum."generateWaves"  # Mode
                  w464 = 0 ("timeout in ms (-1)")
                  w465 = 2.0 items=["Internal"=1.0, "External"=2.0] ("Trigger Source")
                  n126 = Bundle("Enum"=CameraControlTypeDef."Readout Mode", "Trigger Source"=w465, "timeout in ms (-1)"=w464) -> (w469:T15)  [unwired: 1 in]
                  n127 = Enqueue Element(queue=w470, element=w469) -> (queue out=w466:refnum<queue>)  [unwired: 2 in, 2 out]
                  n128 = Bundle("Mode"=w463, "NewVal"=w461) -> (w462:cluster{"Mode":T5, "NewVal":T1})  [unwired: 1 in]
                  n129 = Bundle("Enum"=CameraControlTypeDef."Preview", "Trigger Source"=w465, "timeout in ms (-1)"=w464) -> (w468:T15)  [unwired: 1 in]
                  n130 = Enqueue Element(queue=w460, element=w462) -> ()  [unwired: 2 in, 3 out]
                  n131 = Enqueue Element(queue=w466, element=w468) -> ()  [unwired: 2 in, 3 out]
                  n132 = property on="Microscope Settings" class="Clust (strict)" props=["Value"]() -> ()  [unwired: 2 in, 3 out]
                }
                frame "XYZ" {
                  w473 = 0 ("timeout in ms (-1)")
                  w474 = 2.0 items=["Internal"=1.0, "External"=2.0] ("Trigger Source")
                  n133 = Bundle("Enum"=CameraControlTypeDef."Readout Mode", "Trigger Source"=w474, "timeout in ms (-1)"=w473) -> (w478:T15)  [unwired: 1 in]
                  n134 = Enqueue Element(queue=w479, element=w478) -> (queue out=w477:refnum<queue>)  [unwired: 2 in, 2 out]
                  n135 = Bundle("Enum"=CameraControlTypeDef."Idle", "Trigger Source"=w474, "timeout in ms (-1)"=w473) -> (w476:T15)  [unwired: 1 in]
                  n136 = Enqueue Element(queue=w477, element=w476) -> ()  [unwired: 2 in, 3 out]
                }
                frame "XYZT" {
                }
                frame "XYZC" {
                }
              }
            }
            event "Scan": Value Change {
              w487 = ModeEnum."runWaves"  # Mode
              n137 = event-data() -> ()  [unwired: 1 in, 6 out]
              n138 = Bundle("Mode"=w487, "Value"=w485) -> (w486:cluster{"Mode":T5, "Value":T1})  [unwired: 1 in]
              n139 = Enqueue Element(queue=w483, element=w486) -> (queue out=w484:refnum<queue>)  [unwired: 2 in, 2 out]
            }
            event Timeout {
              n140 = event-data() -> ()  [unwired: 1 in, 3 out]
              n141 = property on="Microscope Settings" class="Clust (strict)"() -> ("Value"=w488:T1)  [unwired: 2 in, 2 out]
            }
          }
        }
        n142 = Merge Errors(w180, w181) -> (w182:errorcluster)
      }
      frame "deinit" {
        n143 = call <vilib>:"DAQmx Stop Task.vi"("task/channels in"=w499) -> ("task out"=w500:refnum<k21>)  [unwired: 13 in, 1 out]
        n144 = call <vilib>:"DAQmx Stop Task.vi"("task/channels in"=w501) -> ("task out"=w502:refnum<k21>)  [unwired: 13 in, 1 out]
        n145 = call <vilib>:"DAQmx Clear Task.vi"("task in"=w500) -> ("error out"=w496:errorcluster)  [unwired: 14 in]
        n146 = call "tm_stopcapture.vi"("error in (no error)"=w511, "Handle in"=w507) -> ("error out"=w514:errorcluster, "Handle out"=w513:u32)  [unwired: 8 in]
        n147 = call <vilib>:"DAQmx Clear Task.vi"("task in"=w502) -> ("error out"=w497:errorcluster)  [unwired: 14 in]
        n148 = call "tm_unpreparecapture.vi"("error in (no error)"=w514, "Handle in"=w513) -> ("error out"=w515:errorcluster, "Handle out"=w512:u32)  [unwired: 8 in]
        n149 = call "tm_closecamera.vi"("error in (no error)"=w515, "Handle in"=w512) -> ("error out"=w516:errorcluster)  [unwired: 9 in]
        n150 = Flush Queue(queue=w489) -> (queue out=w495:refnum<queue>)  [unwired: 1 in, 2 out]
        n151 = call "tm_deinitialize.vi"("error in (no error)"=w516) -> ("error out"=w492:errorcluster)  [unwired: 10 in]
        n152 = Release Queue(queue=w490, error in (no error)=w492) -> (error out=w509:errorcluster)  [unwired: 1 in, 2 out]
        n153 = Release Queue(queue=w495) -> (error out=w498:errorcluster)  [unwired: 2 in, 2 out]
        n154 = Flush Queue(queue=w494, error in (no error)=w492) -> (queue out=w493:refnum<queue>, error out=w491:errorcluster)  [unwired: 1 out]
        n155 = Release Queue(queue=w493, error in (no error)=w491) -> (error out=w508:errorcluster)  [unwired: 1 in, 2 out]
        n156 = Merge Errors(w509, w508, w498, w497, w496) -> (w510:errorcluster)
      }
    }
    n157 = Or(x="stop", y=w22) -> (x .or. y?=w23:bool)
  }
  "error IO" <- w10
  n158 = disable-structure shown="Enabled" {
    frame Disabled {
      # "Parallise decode buffer"
      n159 = call "tm_startcapture_b.vi"() -> ()  [unwired: 10 in, 2 out]
      n160 = call "tm_waitnextframe.vi"() -> ()  [unwired: 8 in, 4 out]
      n161 = call "tm_getframe_a.vi"() -> ()  [unwired: 7 in, 5 out]
    }
    frame Enabled {
    }
  }
